vi "Get ICM File.vi"(8 "error in (no error)":errorcluster, 9 "Re-Init?":bool, 10 "Allow New?":bool, 11 "ICM File In":path) -> (0 "error out":errorcluster, 3 "ICM File":path)   [LabVIEW 2024]
doc: "Get ICM File.vi\n\nThis VI is used to acquire the name of an existing .icm configuration file. If it has been called before, it returns the file it already remembers. (Unless the Re-Init? parameter is True or a new file name is supplied with the ICM File In control.) Otherwise it presents a file dialog for selecting a ICM configuration file.\nThis VI's memory is most useful for the Configuration Editor. In that case, a single file can be selected once and used throughout the program wherever needed. Inside a program that acquires data with the ICM system, each instance of an ICM Driver should be loaded with its own configuration file and should then remember that file name internally for any uses it may have. If this VI is used inside Drivers, then an application that uses more than one Driver could get confused as to which Driver uses which configuration file.\n\nInstrument Communication Module Version 1.0\nJuly, 2017 Original Code Consulting David Thomson\n www.originalcode.com"
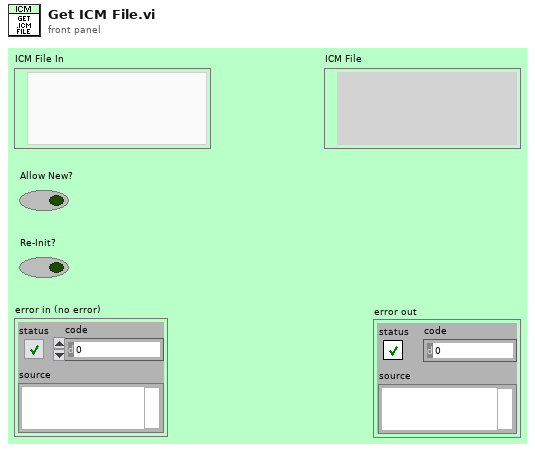
[diagram p1: front panel]
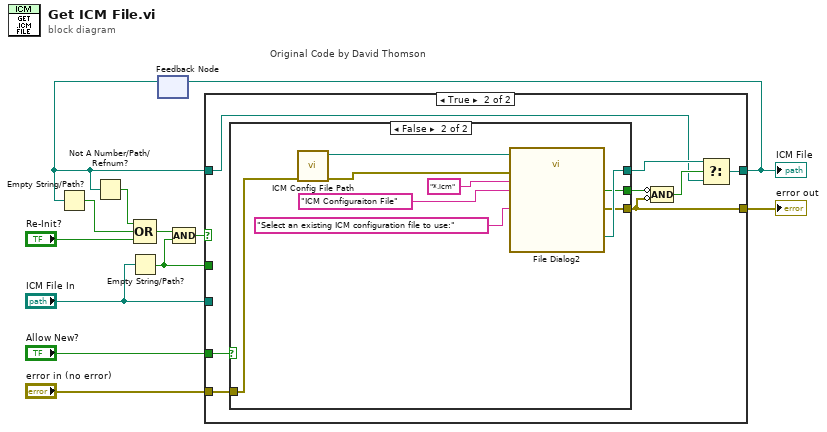
[diagram p0: block diagram]
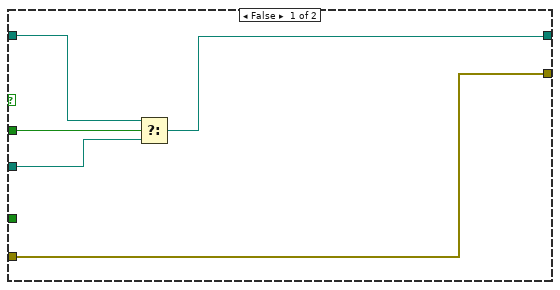
[diagram p2: hidden frame]
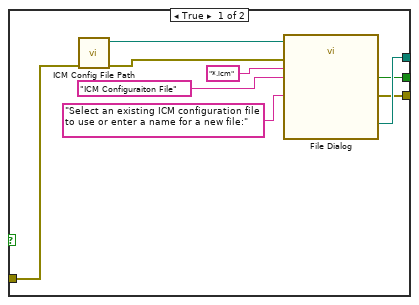
[diagram p3: hidden frame]
diagram:
  n1 = Empty String/Path?(string/path="ICM File In") -> (empty?=w7:bool)
  n2 = feedback #1() -> (w5:path)  [unwired: 1 in]
  n3 = Empty String/Path?(string/path=w5) -> (empty?=w11:bool)
  n4 = Not A Number/Path/Refnum?(number/path/refnum=w5) -> (NaN/Path/Refnum?=w4:bool)
  n5 = Compound Arithmetic op=OR(w4, w11, "Re-Init?") -> (w9:bool)
  n6 = Compound Arithmetic op=AND(w9, w7) -> (w8:bool)
  n7 = case "Original Code by David Thomson" shown="True" w8 {
    tunnel: w5 -> [w15 w19]
    tunnel: [w14 w21] -> w12
    tunnel: w7 -> [w17 _]
    tunnel: "ICM File In" -> [w16 _]
    tunnel: "Allow New?" -> [_ w25]
    tunnel: [w13 w24] -> w2
    tunnel: "error in (no error)" -> [w13 w18]
    frame False {
      n8 = Select(t=w15, s=w17, f=w16) -> (s? t:f=w14:path)
    }
    frame True {
      n9 = case shown="False" w25 {
        tunnel: [w31 w40] -> w20
        tunnel: [w28 w39] -> w24
        tunnel: [w27 w36] -> w23
        tunnel: w18 -> [w26 w35]
        frame True {
          n10 = call "ICM Config File Path.vi"("error in (no error)"=w26) -> ("error out"=w29:errorcluster, "ICM Config Path"=w30:path)  [unwired: 9 in]
          n11 = call "File Dialog"("start path"=w30, "prompt"="Select an existing ICM configuration file to use or enter a name for a new file:", "error in"=w29, "pattern (all files)"="*.icm", "pattern label"="ICM Configuraiton File") -> ("selected path"=w31:path, "cancelled"=w27:bool, "error out"=w28:errorcluster)  [unwired: 7 in, 1 out]
        }
        frame False {
          n12 = call "ICM Config File Path.vi"("error in (no error)"=w35) -> ("error out"=w37:errorcluster, "ICM Config Path"=w38:path)  [unwired: 9 in]
          n13 = call "File Dialog2"("start path"=w38, "prompt"="Select an existing ICM configuration file to use:", "error in"=w37, "pattern (all files)"="*.icm", "pattern label"="ICM Configuraiton File") -> ("selected path"=w40:path, "cancelled"=w36:bool, "error out"=w39:errorcluster)  [unwired: 7 in, 1 out]
        }
      }
      n14 = Compound Arithmetic op=AND(invert w23, invert w24) -> (w22:bool)
      n15 = Select(t=w20, s=w22, f=w19) -> (s? t:f=w21:path)
    }
  }
  "ICM File" <- w12
  "error out" <- w2
  n16 = feedback-in #1(w12) -> ()
